vi "Initialize Messenger.vi"(2 "error in (no error)":errorcluster, 3 "MailboxSize(-1)":i32=-1) -> (0 "error out":errorcluster, 1 "Referencies out":T1)   [LabVIEW 2022 SP3, in "MessengerLib.lvlib"]
doc: "Creates queries for messenger to all modules\nUser interface, Instrument monitor, Magnet controler, Temperature monitor, Temperature controler, Quasi-optical table controler, Microwave controller, Data Aquisition, Modulation monitor, Field monitor, Power monitor, Sample orientation/rotation/angle controler, Specimen Controler (carousel), Reserved (unused)"
uses:
  MessengerLib.lvlib
  Data types/Messenger referencies.ctl
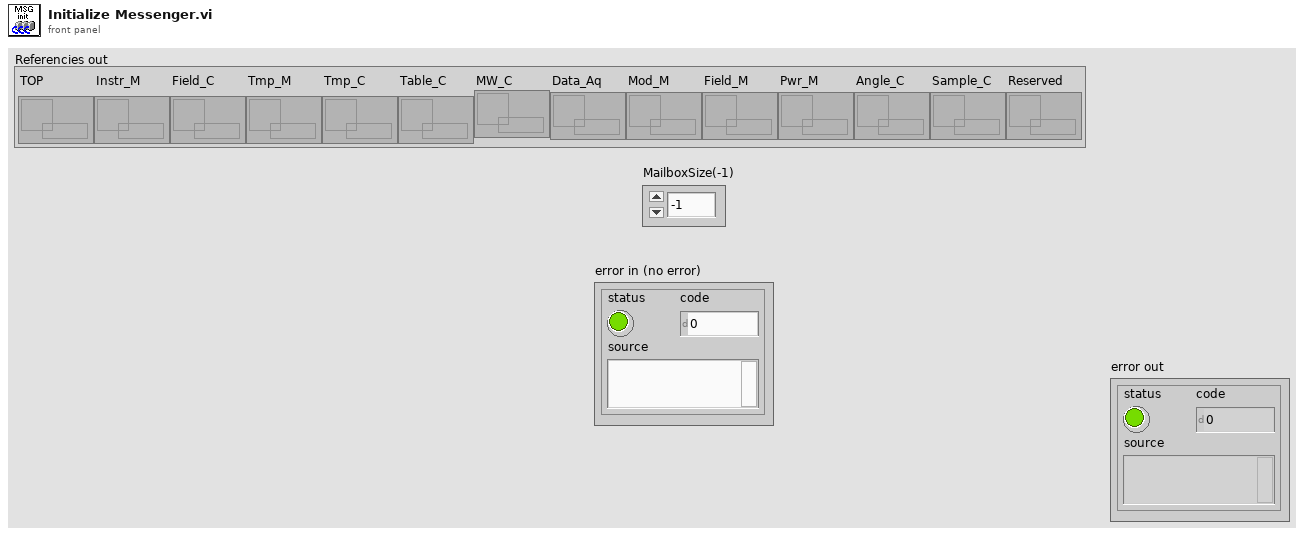
[diagram p1: front panel]
types:
  T1 = typedef "MessengerLib.lvlib/Messenger referencies.ctl" = cluster{"TOP":refnum<queue>, "Instr_M":refnum<queue>, "Field_C":refnum<queue>, "Tmp_M":refnum<queue>, "Tmp_C":refnum<queue>, "Table_C":refnum<queue>, "MW_C":refnum<queue>, "Data_Aq":refnum<queue>, "Mod_M":refnum<queue>, "Field_M":refnum<queue>, "Pwr_M":refnum<queue>, "Angle_C":refnum<queue>, "Sample_C":refnum<queue>, "Reserved":refnum<queue>}
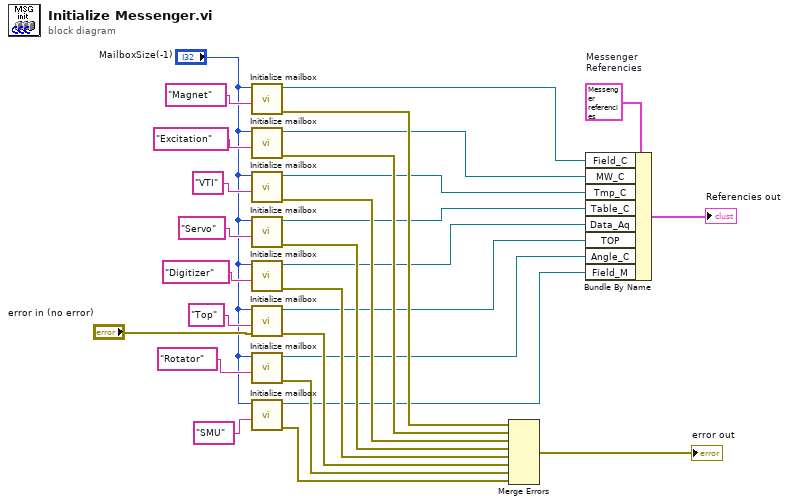
[diagram p0: block diagram]
diagram:
  w28 = T1 {"TOP"=refnum, "Instr_M"=refnum, "Field_C"=refnum, "Tmp_M"=refnum, "Tmp_C"=refnum, "Table_C"=refnum, "MW_C"=refnum, "Data_Aq"=refnum, "Mod_M"=refnum, "Field_M"=refnum, "Pwr_M"=refnum, "Angle_C"=refnum, "Sample_C"=refnum, "Reserved"=refnum}  # Messenger Referencies
  n1 = call "Initialize mailbox.vi"("name (unnamed)"="Magnet", "MailboxSize(-1)"="MailboxSize(-1)") -> ("error out"=w23:errorcluster, "Queue out"=w21:refnum<queue>)  [unwired: 8 in]
  n2 = call "Initialize mailbox.vi"("name (unnamed)"="Excitation", "MailboxSize(-1)"="MailboxSize(-1)") -> ("error out"=w24:errorcluster, "Queue out"=w20:refnum<queue>)  [unwired: 8 in]
  n3 = call "Initialize mailbox.vi"("name (unnamed)"="VTI", "MailboxSize(-1)"="MailboxSize(-1)") -> ("error out"=w25:errorcluster, "Queue out"=w19:refnum<queue>)  [unwired: 8 in]
  n4 = call "Initialize mailbox.vi"("name (unnamed)"="Servo", "MailboxSize(-1)"="MailboxSize(-1)") -> ("error out"=w26:errorcluster, "Queue out"=w18:refnum<queue>)  [unwired: 8 in]
  n5 = call "Initialize mailbox.vi"("name (unnamed)"="Digitizer", "MailboxSize(-1)"="MailboxSize(-1)") -> ("error out"=w27:errorcluster, "Queue out"=w17:refnum<queue>)  [unwired: 8 in]
  n6 = call "Initialize mailbox.vi"("error in"="error in (no error)", "name (unnamed)"="Top", "MailboxSize(-1)"="MailboxSize(-1)") -> ("error out"=w15:errorcluster, "Queue out"=w16:refnum<queue>)  [unwired: 7 in]
  n7 = call "Initialize mailbox.vi"("name (unnamed)"="Rotator", "MailboxSize(-1)"="MailboxSize(-1)") -> ("error out"=w14:errorcluster, "Queue out"=w13:refnum<queue>)  [unwired: 8 in]
  n8 = call "Initialize mailbox.vi"("name (unnamed)"="SMU", "MailboxSize(-1)"="MailboxSize(-1)") -> ("error out"=w10:errorcluster, "Queue out"=w11:refnum<queue>)  [unwired: 8 in]
  n9 = Merge Errors(w23, w24, w25, w26, w27, w15, w14, w10) -> (→"error out":errorcluster)
  n10 = Bundle By Name(cluster=w28, "Field_C"=w21, "MW_C"=w20, "Tmp_C"=w19, "Table_C"=w18, "Data_Aq"=w17, "TOP"=w16, "Angle_C"=w13, "Field_M"=w11) -> (→"Referencies out":T1)
